vi "Decode Disable.vi"(8 "error in (no error)":errorcluster) -> (0 "error out":errorcluster)   [LabVIEW 2019]
uses:
  Globals.vi
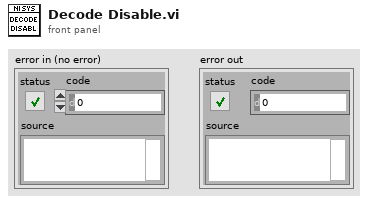
[diagram p1: front panel]
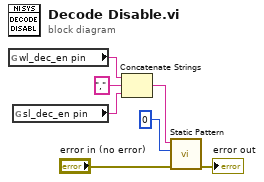
[diagram p0: block diagram]
diagram:
  n1 = global read "Globals.vi" "wl_dec_en pin"() -> (w2:string)
  n2 = global read "Globals.vi" "sl_dec_en pin"() -> (w1:string)
  n3 = Concatenate Strings(w2, "," ("string"), w1) -> (w3:string)
  n4 = call "Static Pattern.vi"("error in (no error)"="error in (no error)", "write data (0x0000)"=u32 0, "channel list (all:\"\")"=w3) -> ("error out"=→"error out":errorcluster)  [unwired: 8 in]
